vi "Create-Destroy.vi"(5 "Username":string, 6 "Password":string, 7 "Address":string, 8 "Error In":errorcluster) -> (0 "Error Out":errorcluster)   [LabVIEW 2018, in "Tests.lvlib" / "Agent.lvlib"]
uses:
  Agent.lvlib
  <vilib>/addons/_JKI Toolkits/Caraya/classes/Test/Test.lvclass
  <vilib>/addons/_JKI Toolkits/Caraya/classes/Assert/Assert.lvclass
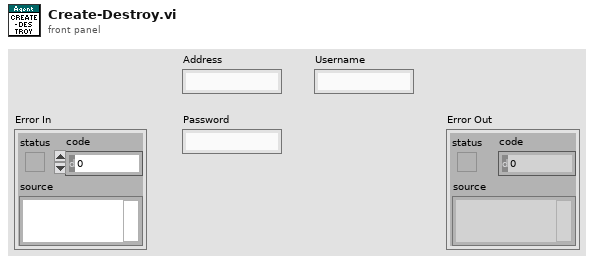
[diagram p1: front panel]
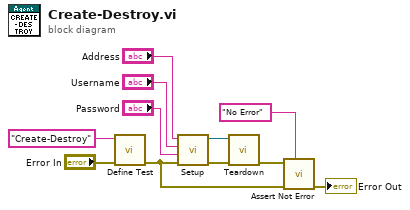
[diagram p0: block diagram]
diagram:
  n1 = call <vilib>:"Define Test.vi"("error in (no error)"="Error In", "Label (VI Title)"="Create-Destroy") -> ("error out"=w5:errorcluster)  [unwired: 9 in]
  n2 = call "Setup.vi"("Error In"=w5, "Password"="Password", "Username"="Username", "Address"="Address") -> ("Error Out"=w6:errorcluster, "Agent"=w7:refnum<class "Agent.lvclass">)  [unwired: 6 in]
  n3 = call "Teardown.vi"("Error In"=w6, "Agent"=w7) -> ("Error Out"=w4:errorcluster)  [unwired: 9 in]
  n4 = call <vilib>:"Assert Not Error.vi"("Label"="No Error", "error in (no error)"=w5, "Not Error?"=w4) -> ("error out"=→"Error Out":errorcluster)  [unwired: 8 in]
